vi "myRIO_BRig_Host_formatData_getHeaders_dataCurrent.vi"() -> (3 "output_stringArray_dataCurrent":string[](array[string]))   [LabVIEW 2014]
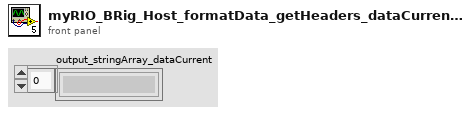
[diagram p1: front panel]
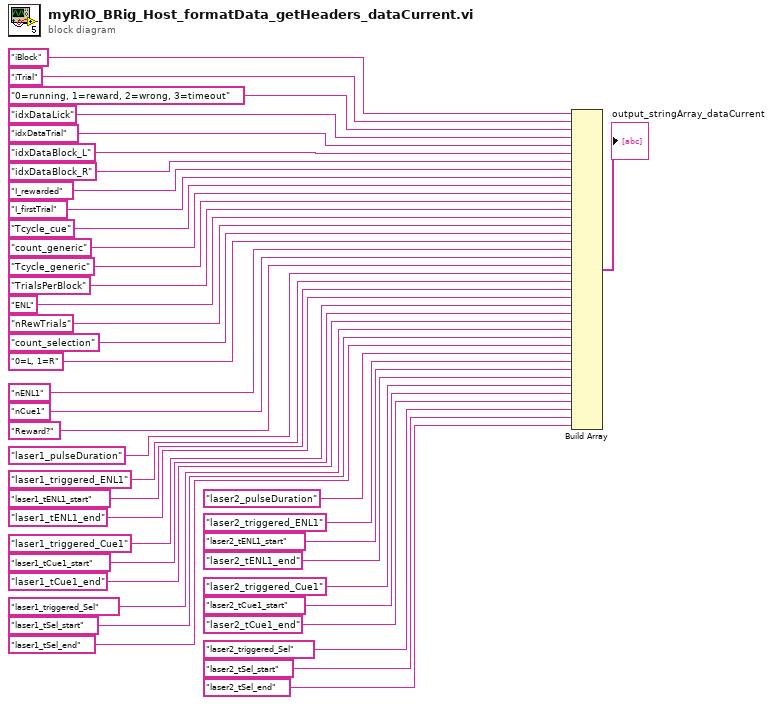
[diagram p0: block diagram]
diagram:
  n1 = Build Array("iBlock", "iTrial", "0=running, 1=reward, 2=wrong, 3=timeout", "idxDataLick", "idxDataTrial", "idxDataBlock_L", "idxDataBlock_R", "I_rewarded", "I_firstTrial", "Tcycle_cue", "count_generic", "Tcycle_generic", "TrialsPerBlock", "ENL", "nRewTrials", "count_selection", "0=L, 1=R", "nENL1", "nCue1", "Reward?", "laser1_pulseDuration", "laser1_triggered_ENL1", "laser1_tENL1_start", "laser1_tENL1_end", "laser1_triggered_Cue1", "laser1_tCue1_start", "laser1_tCue1_end", "laser1_triggered_Sel", "laser1_tSel_start", "laser1_tSel_end", "laser2_pulseDuration", "laser2_triggered_ENL1", "laser2_tENL1_start", "laser2_tENL1_end", "laser2_triggered_Cue1", "laser2_tCue1_start", "laser2_tCue1_end", "laser2_triggered_Sel", "laser2_tSel_start", "laser2_tSel_end") -> (→"output_stringArray_dataCurrent":string[])
